vi "ExampleQueryServer.vi"() -> ()   [LabVIEW 2019]
uses:
  VIs/QueryServer_gRPCid.ctl
panel:
  in  "stop":bool
  in  "Server Address":string
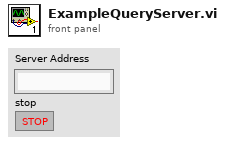
[diagram p1: front panel]
types:
  T1 = typedef "QueryServer_gRPCid.ctl" = cluster{"ID":u64}
  T2 = cluster{"event":refnum<user-event>, "event":refnum<user-event>, "event":refnum<user-event>}
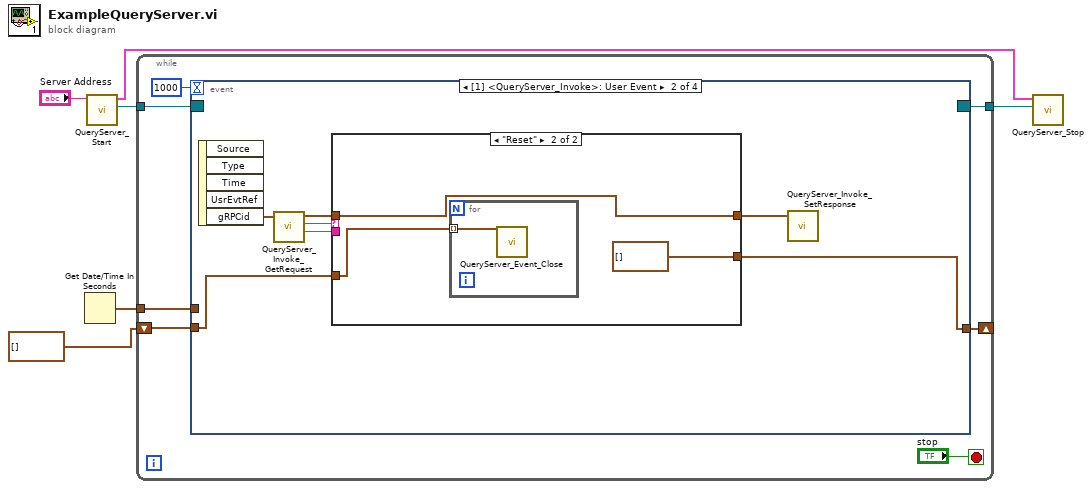
[diagram p0: block diagram]
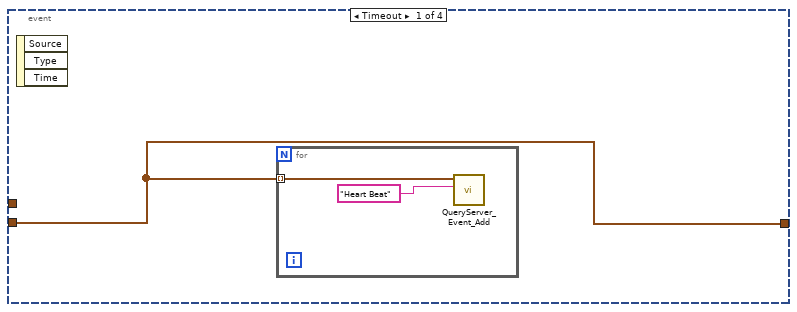
[diagram p2: hidden frame]
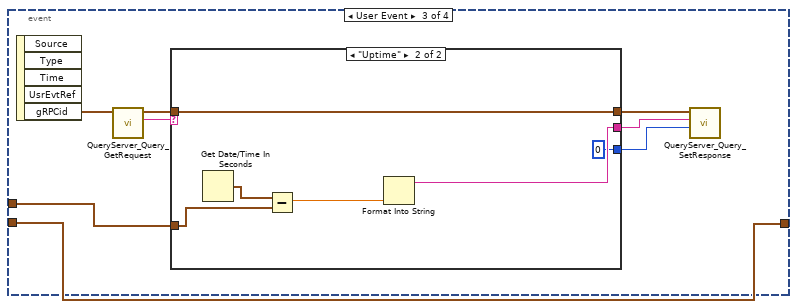
[diagram p4: hidden frame]
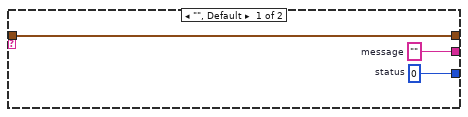
[diagram p5: hidden frame]
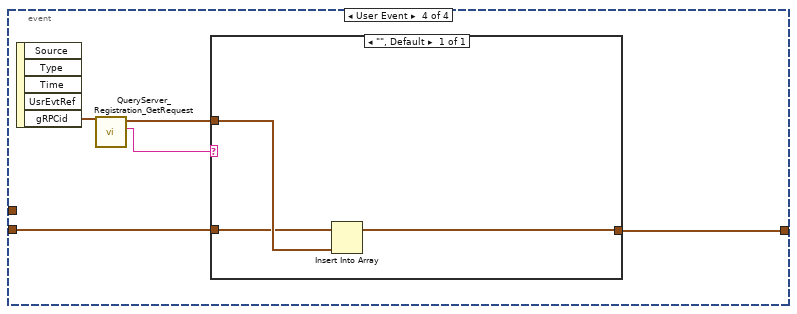
[diagram p6: hidden frame]
diagram:
  n1 = Get Date/Time In Seconds() -> (seconds since 1Jan1904=w2:timestamp)
  n2 = call "QueryServer_Start.vi"("Server Address"="Server Address") -> ("Event Registration Refnum"=w5:refnum<event-registration>, "Server Events"=w3:T2)  [unwired: 7 in, 1 out]
  n3 = while {
    tunnel: w5 -> [w12]
    tunnel: [w11] -> w4
    tunnel: w2 -> [w10]
    shift-right: [w8] -> _
    shift-left: T1[] [] -> [w7]
    stop <- "stop" stop-if-true
    n4 = event shown="[1] <QueryServer_Invoke>: User Event" {
      selector: w12 -> [_ _ _ _]
      dyn-events: [_ _ _ _] -> w11
      timeout: 1000 -> [_ _ _ _]
      tunnel: w10 -> [_ _ w31 _]
      tunnel: [w14 w17 w30 w48] -> w8
      tunnel: w7 -> [w14 w18 w30 w47]
      event Timeout {
        n5 = event-data() -> ()  [unwired: 1 in, 3 out]
        n6 = for {
          tunnel: w14 -> [w16] mode=indexing
          n7 = call "QueryServer_Event_Add.vi"("eventdata"="Heart Beat", "gRPCid"=w16) -> ()  [unwired: 8 in, 2 out]
        }
      }
      event User Event {
        n8 = event-data() -> ("gRPCid"=w23:T1)  [unwired: 1 in, 4 out]
        n9 = call "QueryServer_Invoke_GetRequest.vi"("gRPCid"=w23) -> ("parameter"=w19:string, "command"=w22:string, "gRPCid out"=w21:T1)  [unwired: 5 in, 1 out]
        n10 = case shown="\"Reset\"" w22 {
          tunnel: w21 -> [w25 w26]
          tunnel: [w25 w26] -> w20
          tunnel: w19 -> [_ _]
          tunnel: w18 -> [w24 w28]
          tunnel: [w24 T1[] []] -> w17
          frame "", Default {
          }
          frame "Reset" {
            n11 = for {
              tunnel: w28 -> [w29] mode=indexing
              n12 = call "QueryServer_Event_Close.vi"("gRPCid"=w29) -> ()  [unwired: 9 in, 1 out]
            }
          }
        }
        n13 = call "QueryServer_Invoke_SetResponse.vi"("gRPCid"=w20) -> ()  [unwired: 9 in, 1 out]
      }
      event User Event {
        n14 = event-data() -> ("gRPCid"=w37:T1)  [unwired: 1 in, 4 out]
        n15 = call "QueryServer_Query_GetRequest.vi"("gRPCid"=w37) -> ("gRPCid out"=w35:T1, "query"=w36:string)  [unwired: 7 in, 1 out]
        n16 = case shown="\"Uptime\"" w36 {
          tunnel: w35 -> [w40 w42]
          tunnel: [w40 w42] -> w34
          tunnel: [w39 w43] -> w33
          tunnel: [w38 0 ("status")] -> w32
          tunnel: w31 -> [_ w45]
          frame "", Default {
            w38 = 0  # status
            w39 = ""  # message
          }
          frame "Uptime" {
            n17 = Get Date/Time In Seconds() -> (seconds since 1Jan1904=w46:timestamp)
            n18 = Subtract(x=w46, y=w45) -> (x-y=w44:dbl)
            n19 = Format Into String(w44) -> (resulting string=w43:string)  [unwired: 3 in, 1 out]
          }
        }
        n20 = call "QueryServer_Query_SetResponse.vi"("gRPCid"=w34, "message"=w33, "status"=w32) -> ()  [unwired: 7 in, 1 out]
      }
      event User Event {
        n21 = event-data() -> ("gRPCid"=w51:T1)  [unwired: 1 in, 4 out]
        n22 = call "QueryServer_Registration_GetRequest.vi"("gRPCid"=w51) -> ("gRPCid out"=w49:T1, "eventname"=w50:string)  [unwired: 7 in, 1 out]
        n23 = case shown="\"\", Default" w50 {
          tunnel: w49 -> [w54]
          tunnel: [w53] -> w48
          tunnel: w47 -> [w52]
          frame "", Default {
            n24 = Insert Into Array(array=w52, new element=w54) -> (w53:T1[])  [unwired: 1 in]
          }
        }
      }
    }
  }
  n25 = call "QueryServer_Stop.vi"("Server Events"=w3, "Event Registration Refnum"=w4) -> ()  [unwired: 8 in, 1 out]
